vi "MGI Scan From String (DBL[]).vi"(7 "format string":string="%g", 8 "Default DBL[]":dbl[](array[numeric]), 9 "error in (no error)":errorcluster, 11 "String[]":string[](array[string])) -> (0 "DBL[] Out":dbl[](array[numeric]), 1 "error out":errorcluster)   [LabVIEW 2016]
doc: "This PolyVI handles scan from string for special datatypes.\n\nAuthored by Shawn Walpole\nsupport@mooregoodideas.com\nwww.mooregoodideas.com\n\nCopyright (c) 2010, Moore Good Ideas, Inc.\n\nAll rights reserved.\n\nRedistribution and use in source and binary forms, with or without modification, are permitted provided that the following conditions are met:\n\n * Redistributions of source code must retain the above copyright notice, this list of conditions and the following disclaimer.\n * Redistributions in binary form must reproduce the above copyright notice, this list of conditions and the following disclaimer in the documentation and/or other materials provided with the distribution.\n * Neither the name of Moore Good Ideas, Inc. nor the names of its contributors may be used to endorse or promote products derived from this software without specific prior written permission.\n\nTHIS SOFTWARE IS PROVIDED BY THE COPYRIGHT HOLDERS AND CONTRIBUTORS \"AS IS\" AND ANY EXPRESS OR IMPLIED WARRANTIES, INCLUDING, BUT NOT LIMITED TO, THE IMPLIED WARRANTIES OF MERCHANTABILITY AND FITNESS FOR A PARTICULAR PURPOSE ARE DISCLAIMED. IN NO EVENT SHALL THE COPYRIGHT OWNER OR CONTRIBUTORS BE LIABLE FOR ANY DIRECT, INDIRECT, INCIDENTAL, SPECIAL, EXEMPLARY, OR CONSEQUENTIAL DAMAGES (INCLUDING, BUT NOT LIMITED TO, PROCUREMENT OF SUBSTITUTE GOODS OR SERVICES; LOSS OF USE, DATA, OR PROFITS; OR BUSINESS INTERRUPTION) HOWEVER CAUSED AND ON ANY THEORY OF LIABILITY, WHETHER IN CONTRACT, STRICT LIABILITY, OR TORT (INCLUDING NEGLIGENCE OR OTHERWISE) ARISING IN ANY WAY OUT OF THE USE OF THIS SOFTWARE, EVEN IF ADVISED OF THE POSSIBILITY OF SUCH DAMAGE."
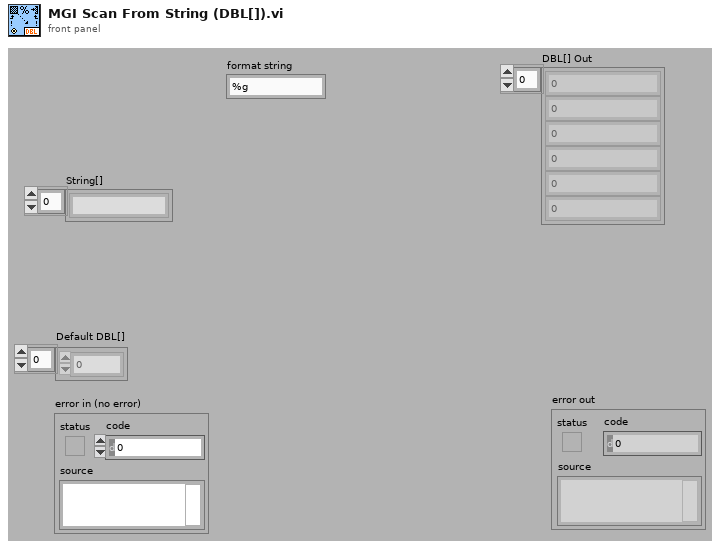
[diagram p1: front panel]
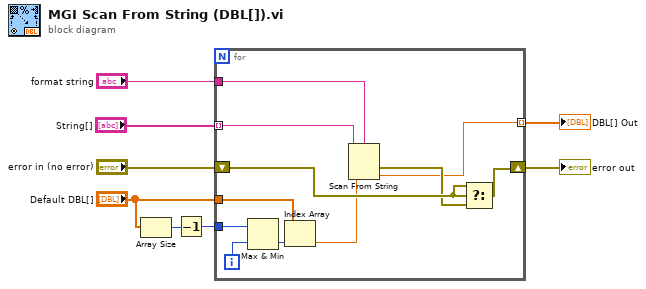
[diagram p0: block diagram]
diagram:
  n1 = Array Size(array="Default DBL[]") -> (size(s)=w5:i32)
  n2 = Decrement(x=w5) -> (x-1=w4:i32)
  n3 = for {
    tunnel: "String[]" -> [w12] mode=indexing
    tunnel: "Default DBL[]" -> [w17]
    tunnel: "format string" -> [w15]
    tunnel: [w9] -> w7 mode=indexing
    tunnel: w4 -> [w18]
    shift-right: [w13] -> w3
    shift-left: "error in (no error)" -> [w14]
    i -> [w19]
    n4 = Max & Min(x=w18, y=w19) -> (min(x,y)=w16:i32)  [unwired: 1 out]
    n5 = Index Array(array=w17, index=w16) -> (element=w10:dbl)
    n6 = Scan From String(format string=w15, input string=w12, default 1=w10) -> (error out=w11:errorcluster, output 1=w9:dbl)  [unwired: 2 in, 2 out]
    n7 = Select(t=w14, s=w14, f=w11) -> (s? t:f=w13:errorcluster)
  }
  "DBL[] Out" <- w7
  "error out" <- w3
